vi "Pulse Attribute, Set Input Parms.vi"(4 "Average Size":dbl=10.0, 5 "Resistance (ohms)":dbl=500.0 format="%.1f", 6 "error in":errorcluster, 9 "waveform":waveform(dbl)={"t0"=timestamp(3472747248.0780005 s since 1904-01-01), "dt"=2e-06, "Y"=[]}) -> (0 "error out":errorcluster, 3 "waveform out":waveform(dbl)={"t0"=timestamp(0 s since 1904-01-01), "dt"=nan, "Y"=[]})   [LabVIEW 2010]
doc: "This function sets waveform input parameters as waveform attributes."
panel:
  out "Number of Samples":dbl=nan min=3.0 format="%.3f"
  out "dt (us)":dbl=nan min=3.0 format="%.3f"
  out "Sample Frequency (MHz)":dbl=nan min=3.0 format="%.3f"
  # "Sample Interval"
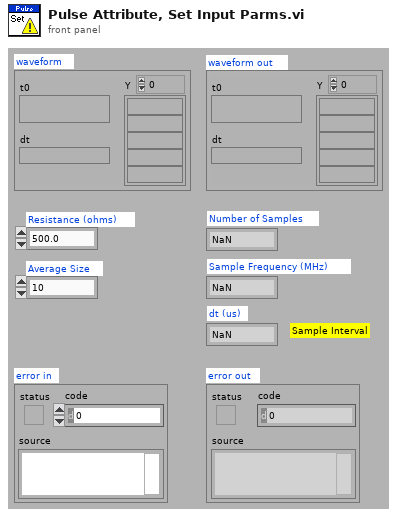
[diagram p1: front panel]
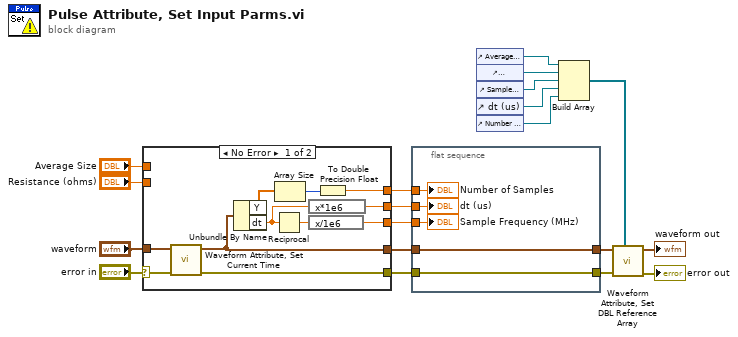
[diagram p0: block diagram]
diagram:
  n1 = case shown="No Error" "error in" {
    selector: "error in" -> [w23 w31]
    tunnel: [w30 _] -> w19
    tunnel: "waveform" -> [w21 _]
    tunnel: "Average Size" -> [_ _]
    tunnel: [w20 _] -> w16
    tunnel: [w22 w31] -> w14
    tunnel: [w27 _] -> w7
    tunnel: [w24 _] -> w5
    tunnel: "Resistance (ohms)" -> [_ _]
    frame No Error {
      n2 = call "Waveform Attribute, Set Current Time.vi"("error in"=w23, "waveform"=w21) -> ("error out"=w22:errorcluster, "waveform out"=w20:waveform(dbl))  [unwired: 4 in, 2 out]
      n3 = Unbundle By Name(w20) -> ("Y"=w26:dbl[], "dt"=w28:dbl)
      n4 = Reciprocal(x=w28) -> (1/x=w29:dbl)
      n5 = Array Size(array=w26) -> (size(s)=w25:i32)
      n6 = expression code="x*1e6"(w28) -> (w27:dbl)
      n7 = expression code="x/1e6"(w29) -> (w30:dbl)
      n8 = To Double Precision Float(number=w25) -> (double precision float=w24:dbl)
    }
    frame Error {
    }
  }
  n9 = flat-sequence {
    tunnel: w19 -> [w36]
    tunnel: w16 -> [w34]
    tunnel: w14 -> [w35]
    tunnel: [w35] -> w13
    tunnel: [w34] -> w8
    tunnel: w7 -> [w33]
    tunnel: w5 -> [w32]
    frame #0 {
      "Sample Frequency (MHz)" <- w36
      "dt (us)" <- w33
      "Number of Samples" <- w32
    }
  }
  n10 = control-ref of="Average Size"() -> (w2:refnum<vi>)
  n11 = control-ref of="Resistance (ohms)"() -> (w1:refnum<vi>)
  n12 = control-ref of="Sample Frequency (MHz)"() -> (w11:refnum<vi>)
  n13 = control-ref of="dt (us)"() -> (w6:refnum<vi>)
  n14 = control-ref of="Number of Samples"() -> (w4:refnum<vi>)
  n15 = Build Array(w2, w1, w11, w6, w4) -> (w10:refnum<vi>[])
  n16 = call "Waveform Attribute, Set DBL Reference Array.vi"("Refnum Array"=w10, "error in"=w13, "waveform"=w8) -> ("error out"=→"error out":errorcluster, "waveform out"=→"waveform out":waveform(dbl))  [unwired: 5 in]
